vi "Pre-Actor.vi"(8 "error in (no error)":errorcluster, 11 "Analog-Output in":refnum<class "Analog-Output.lvclass">) -> (0 "error out":errorcluster, 3 "Analog-Output out":refnum<class "Analog-Output.lvclass">)   [LabVIEW 2019, in "Analog-Output.lvlib" / "Analog-Output.lvclass"]
doc: "This override VI is to provide the means for children classes to perform application specific post launch initialization functions that must be performed *prior* to calling the actor. \n\n***DO NOT USE THE CHECK FOR FAULT ROUTINE HERE***"
uses:
  Library/Analog-Output.lvclass
  Library/Analog-Output.lvclass/Analog-Output.ctl
  builds/Instruments/Instruments.lvlibp/Library/Instruments.lvclass
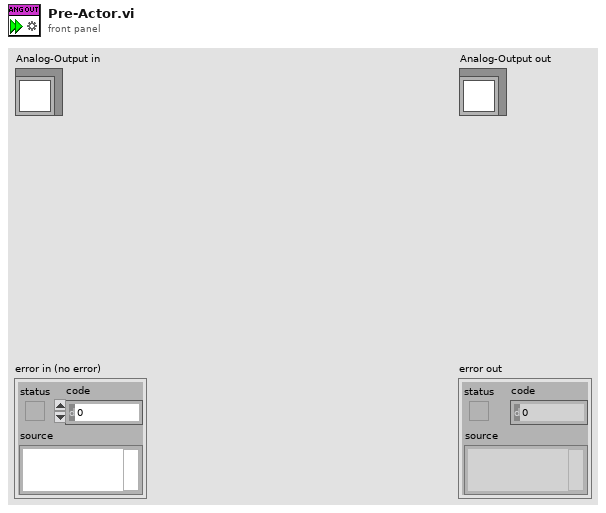
[diagram p1: front panel]
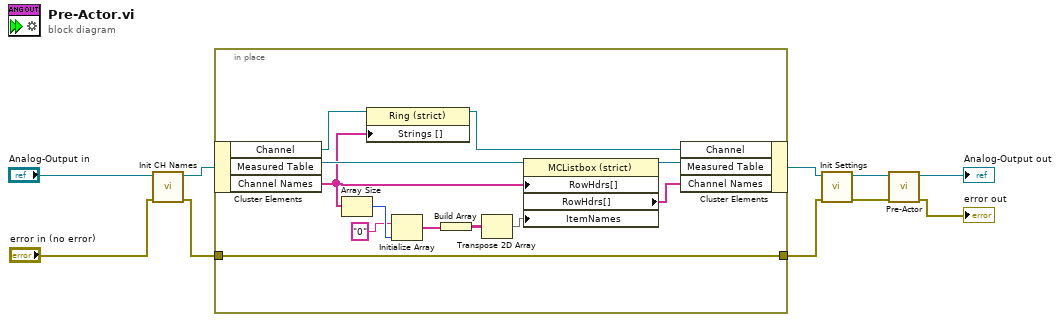
[diagram p0: block diagram]
diagram:
  n1 = call "Init CH Names.vi"("error in (no error)"="error in (no error)", "Analog-Output in"="Analog-Output in") -> ("error out"=w5:errorcluster, "Analog-Output out"=w8:refnum<class "Analog-Output.lvclass">)  [unwired: 8 in]
  n2 = in-place {
    in-place-border: w5 -> [w19]
    in-place-border: [w19] -> w1
    n3 = in-place-cluster #1(w8) -> ("Channel"=w18:refnum<vi>, "Measured Table"=w22:refnum<vi>, "Channel Names"=w16:string[])
    n4 = Array Size(array=w16) -> (size(s)=w15:i32)
    n5 = property class="Ring (strict)"(reference=w18, "Strings []"=w16) -> (reference out=w17:refnum<vi>)  [unwired: 1 in, 1 out]
    n6 = Initialize Array("0", w15) -> (w13:string[])
    n7 = Build Array(w13) -> (w11:string[][])
    n8 = Transpose 2D Array(2D array=w11) -> (transposed array=w12:string[][])
    n9 = property class="MCListbox (strict)"(reference=w22, "RowHdrs[]"=w16, "ItemNames"=w12) -> (reference out=w21:refnum<vi>, "RowHdrs[]"=w20:string[])  [unwired: 1 in, 1 out]
    n10 = in-place-cluster #1("Channel"=w17, "Measured Table"=w21, "Channel Names"=w20) -> (w2:refnum<class "Analog-Output.lvclass">)
  }
  n11 = call "Init Settings.vi"("error in"=w1, "Analog-Output in"=w2) -> ("error out"=w3:errorcluster, "Analog-Output out"=w4:refnum<class "Analog-Output.lvclass">)  [unwired: 8 in]
  n12 = call-parent "Pre-Actor.vi"("error in (no error)"=w3, "Instruments in"=w4) -> ("error out"=→"error out":errorcluster, "Instruments out"=→"Analog-Output out":refnum<class "Analog-Output.lvclass">)  [unwired: 8 in]
